vi "AI engedélyezés refresh.vi"(8 "error in (no error)":errorcluster, 10 "AI engedélyezés":bool, 11 "Message Queues in":T1) -> (0 "error out":errorcluster)   [LabVIEW 2014]
uses:
  support/Message Queue/All Message Queues.ctl
  support/Message Queue/Message Cluster.ctl
  Analog Input Cluster.ctl
  Analog Result Cluster.ctl
  support/Message Queue/Lossy Enqueue Message (Single).vi
  support/Message Queue/Message Queue.lvlib
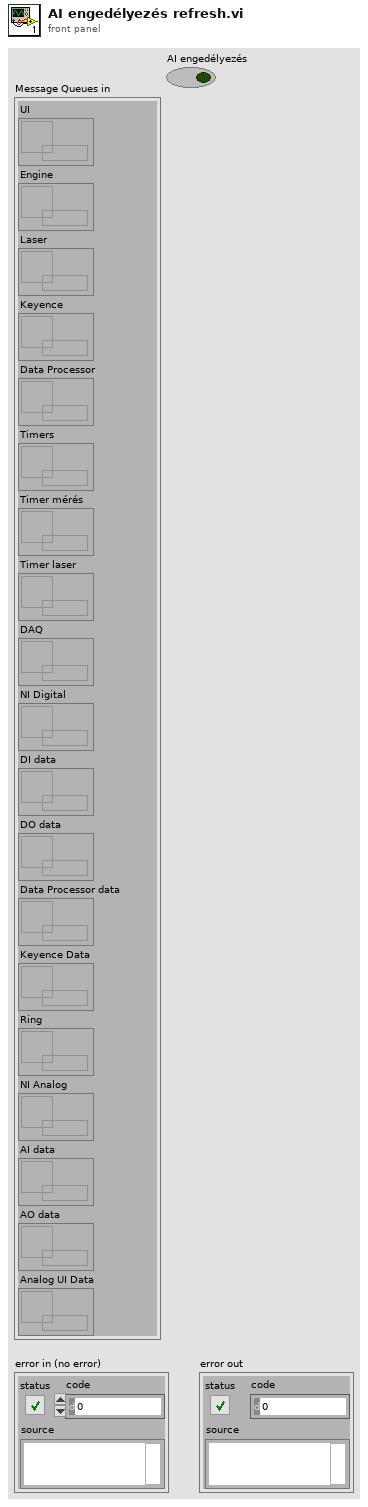
[diagram p1: front panel]
types:
  T1 = typedef "Message Queue.lvlib/All Message Queues.ctl" = cluster{"UI":refnum<queue>, "Engine":refnum<queue>, "Laser":refnum<queue>, "Keyence":refnum<queue>, "Data Processor":refnum<queue>, "Timers":refnum<queue>, "Timer mérés":refnum<queue>, "Timer laser":refnum<queue>, "DAQ":refnum<queue>, "NI Digital":refnum<queue>, "DI data":refnum<queue>, "DO data":refnum<queue>, "Data Processor data":refnum<queue>, "Keyence Data":refnum<queue>, "Ring":refnum<queue>, "NI Analog":refnum<queue>, "AI data":refnum<queue>, "AO data":refnum<queue>, "Analog UI Data":refnum<queue>}
  T2 = typedef "Analog Input Cluster.ctl" = cluster{"NI-6221":cluster{"Sensor":dbl, "Uref":dbl, "Temperature":dbl, "Uisol":dbl, "NTC":dbl, "U48":dbl, "U15":dbl}, "Analog Result":T3, "AI engedélyezés":bool, "dU":dbl[]}
  T3 = typedef "Analog Result Cluster.ctl" = cluster{"Szenzor ellenállás":dbl, "NTC ellenállás":dbl, "Szigetelési ellenállás":dbl, "Hõmérséklet":dbl, "48V":dbl, "15V":dbl, "Elvárt NTC ellenállás":dbl, "Számolt NTC hõmérséklet":dbl}
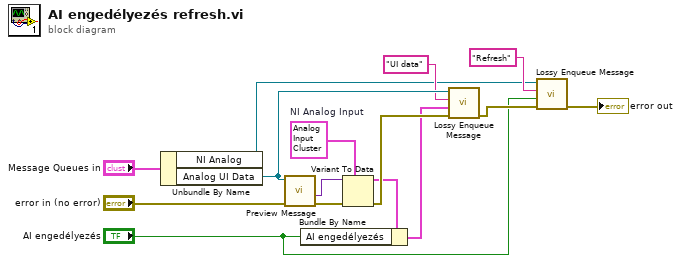
[diagram p0: block diagram]
diagram:
  w7 = T2 {"NI-6221"={"Sensor"=0.0, "Uref"=0.0, "Temperature"=0.0, "Uisol"=0.0, "NTC"=0.0, "U48"=0.0, "U15"=0.0}, "Analog Result"={"Szenzor ellenállás"=0.0, "NTC ellenállás"=0.0, "Szigetelési ellenállás"=0.0, "Hõmérséklet"=0.0, "48V"=0.0, "15V"=0.0, "Elvárt NTC ellenállás"=0.0, "Számolt NTC hõmérséklet"=0.0}, "AI engedélyezés"=FALSE, "dU"=[]}  # NI Analog Input
  n1 = Unbundle By Name("Message Queues in") -> ("NI Analog"=w2:refnum<queue>, "Analog UI Data"=w6:refnum<queue>)
  n2 = call "Preview Message.vi"("error in (no error)"="error in (no error)", "Message Queue"=w6) -> ("error out"=w12:errorcluster, "Message Data"=w5:variant)  [unwired: 5 in, 3 out]
  n3 = Variant To Data(error in=w12, type=w7, Variant=w5) -> (data=w8:T2, error out=w13:errorcluster)
  n4 = Bundle By Name(cluster=w8, "AI engedélyezés"="AI engedélyezés") -> (w3:T2)
  n5 = call-poly "Lossy Enqueue Message.vi"("error in (no error)"=w13, "Message Data"=w3, "Message"="UI data", "Message Queue"=w6) -> ("error out"=w14:errorcluster)  [unwired: 6 in, 1 out]
  n6 = call-poly "Lossy Enqueue Message.vi"("error in (no error)"=w14, "Message Data"="AI engedélyezés", "Message"="Refresh", "Message Queue"=w2) -> ("error out"=→"error out":errorcluster)  [unwired: 6 in, 1 out]
